vi "Slewing Test.vi"(8 "error in (no error)":errorcluster, 11 "Context in":refnum<class "Context.lvclass">) -> (0 "error out":errorcluster, 3 "Context out":refnum<class "Context.lvclass">)   [LabVIEW 2016, in "Context.lvclass"]
uses:
  Context.lvclass
  Context.lvclass/Context.ctl
  States/State/State.lvclass
  Model/Model/Model.lvclass
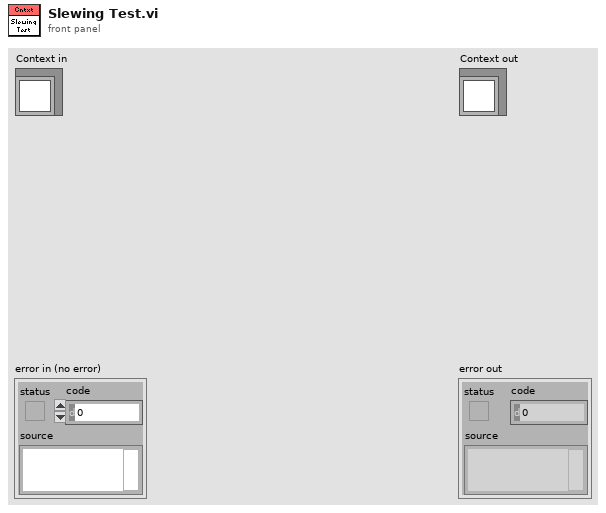
[diagram p1: front panel]
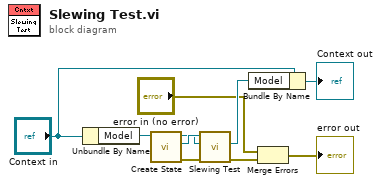
[diagram p0: block diagram]
diagram:
  n1 = Unbundle By Name("Context in") -> ("Model"=w10:refnum<class "Model.lvclass">)
  n2 = call "Create State.vi"("Model in"=w10) -> ("error out"=w4:errorcluster, "State"=w9:refnum<class "State.lvclass">, "Model out"=w8:refnum<class "Model.lvclass">)  [unwired: 8 in]
  n3 = call-dynamic "Slewing Test.vi"("error in (no error)"=w4, "Model in"=w8, "State in"=w9) -> ("error out"=w3:errorcluster, "Model out"=w7:refnum<class "Model.lvclass">)  [unwired: 6 in, 1 out]
  n4 = Bundle By Name(cluster="Context in", "Model"=w7) -> (→"Context out":refnum<class "Context.lvclass">)
  n5 = Merge Errors("error in (no error)", w3) -> (→"error out":errorcluster)
